vi "Full_Client_Name.vi"() -> (0 "Client Name":string)   [LabVIEW 2021]
uses:
  Anemometry/Anemometry Sub Vis/Globals/Preference_global.vi
  Anemometry/Anemometry Sub Vis/Globals/Dynamic_call_global.ph.vi
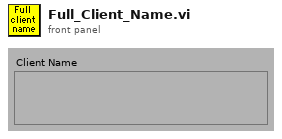
[diagram p1: front panel]
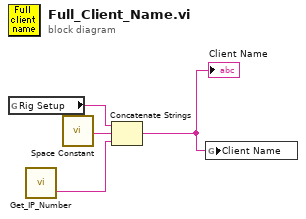
[diagram p0: block diagram]
diagram:
  n1 = global read "Preference_global.vi" "Rig Setup"() -> (w4:string)
  n2 = call "Get_IP_Number.vi"() -> ("bestAvailableName"=w2:string)  [unwired: 1 out]
  n3 = call <vilib>:"Space Constant.vi"() -> ("String"=w3:string)
  n4 = Concatenate Strings(w4, w3, w2) -> (w1:string)
  "Client Name" <- w1
  n5 = global write "Dynamic_call_global.ph.vi" "Client Name"(w1) -> ()
